vi "Filter Remote Sessions.vi"(8 "error in":errorcluster, 10 "Detected Sessions":string[](array[string]), 11 "Windows TCP Ports":string[](array[string])) -> (0 "error out":errorcluster, 3 "Filtered Remote Sessions":string[][](array[string]))   [LabVIEW 2024, in "Session Scanner.lvlib"]
uses:
  Session Scanner.lvlib
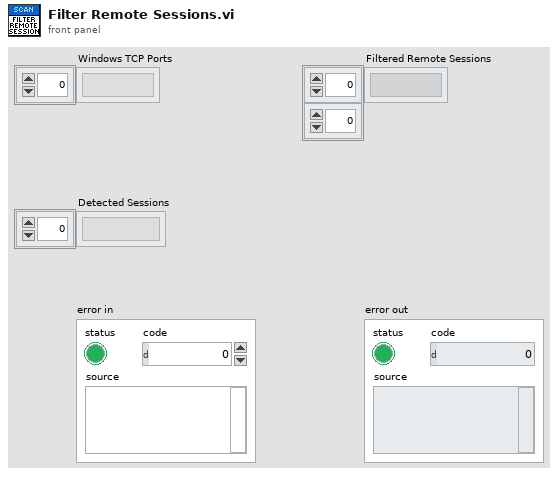
[diagram p1: front panel]
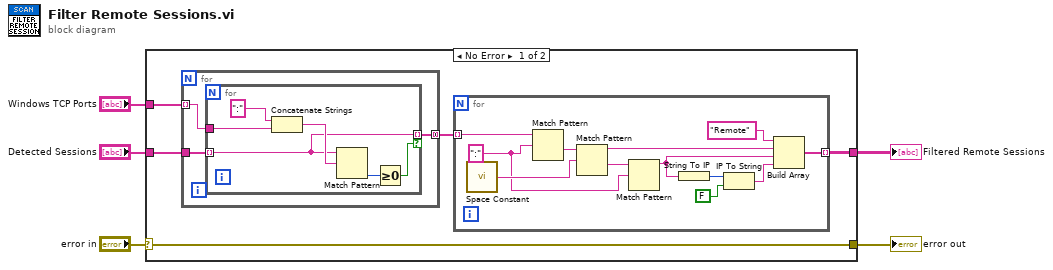
[diagram p0: block diagram]
diagram:
  n1 = case shown="No Error" "error in" {
    selector: "error in" -> [w6 w32]
    tunnel: "Windows TCP Ports" -> [w10 _]
    tunnel: "Detected Sessions" -> [w9 _]
    tunnel: [w7 _] -> w3
    tunnel: [w6 w32] -> w1
    frame No Error {
      n2 = for {
        tunnel: w9 -> [w13]
        tunnel: w10 -> [w12] mode=indexing
        tunnel: [w11] -> w8 mode=concatenating
        n3 = for {
          tunnel: w13 -> [w15] mode=indexing
          tunnel: w12 -> [w18]
          tunnel: [w15] -> w11 mode=indexing if=w14
          n4 = Concatenate Strings(":" ("string"), w18) -> (w17:string)
          n5 = Match Pattern(string=w15, regular expression=w17) -> (offset past match=w16:i32)  [unwired: 1 in, 3 out]
          n6 = Greater Or Equal To 0?(x=w16) -> (x >= 0?=w14:bool)
        }
      }
      n7 = for {
        tunnel: w8 -> [w31] mode=indexing
        tunnel: [w20] -> w7 mode=indexing
        w25 = ":" ("regular expression")
        n8 = call <vilib>:"Space Constant.vi"() -> ("String"=w29:string)
        n9 = Match Pattern(string=w31, regular expression=w25) -> (after substring=w30:string)  [unwired: 1 in, 3 out]
        n10 = Match Pattern(string=w30, regular expression=w29) -> (before substring=w23:string, after substring=w28:string)  [unwired: 1 in, 2 out]
        n11 = Match Pattern(string=w28, regular expression=w25) -> (before substring=w22:string)  [unwired: 1 in, 3 out]
        n12 = String To IP(1:w22) -> (0:w27:u32)
        n13 = IP To String(1:FALSE ("dot notation? (F)"), 2:w27) -> (0:w21:string)
        n14 = Build Array("Remote", w23, w22, w21) -> (w20:string[])
      }
    }
    frame Error {
    }
  }
  "error out" <- w1
  "Filtered Remote Sessions" <- w3
